vi "AmplifySignal4IMG.vi"(8 "error in (no error)":errorcluster, 11 "resampled waveform in":waveform(dbl)) -> (0 "error out":errorcluster, 3 "Waveform":waveform(dbl))   [LabVIEW 2018]
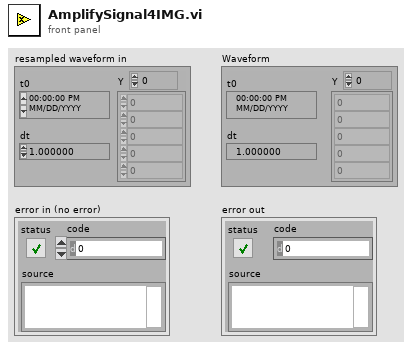
[diagram p1: front panel]
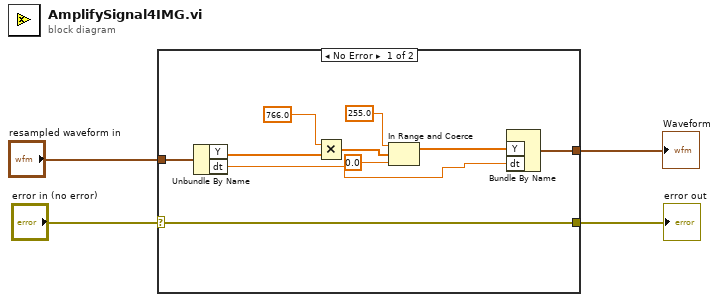
[diagram p0: block diagram]
diagram:
  n1 = case shown="No Error" "error in (no error)" {
    selector: "error in (no error)" -> [w5 w15]
    tunnel: "resampled waveform in" -> [w14 w16]
    tunnel: [w6 w16] -> w2
    tunnel: [w5 w15] -> w4
    frame No Error {
      n2 = Unbundle By Name(w14) -> ("Y"=w11:dbl[], "dt"=w7:dbl)
      n3 = Multiply(x=766.0, y=w11) -> (x*y=w10:dbl[])
      n4 = In Range and Coerce(upper limit=255.0, x=w10, lower limit=0.0) -> (coerced(x)=w8:dbl[])  [unwired: 1 out]
      n5 = Bundle By Name("Y"=w8, "dt"=w7) -> (w6:waveform(dbl))  [unwired: 1 in]
    }
    frame Error {
    }
  }
  "error out" <- w4
  "Waveform" <- w2
